vi "CRYProject Editor PIC Generater WSYS.vi"() -> (2 "sData_Out":string)   [LabVIEW 2013]
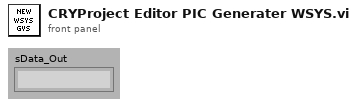
[diagram p1: front panel]
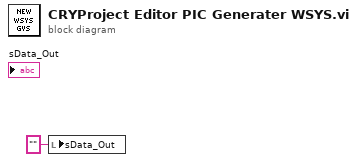
[diagram p0: block diagram]
diagram:
  n1 = local write "sData_Out"("" ("sData_Out")) -> ()
